vi "test Acyclic Loopback Selective Triggers.vi"(8 "error in":errorcluster, 11 "TestCase in":refnum<class "Single Board Loopback.lvclass">) -> (0 "error out":errorcluster, 3 "TestCase out":refnum<class "Single Board Loopback.lvclass">)   [LabVIEW 2020, in "Single Board Loopback.lvclass"]
uses:
  Single Board Loopback.lvclass
  <vilib>/addons/_JKI Toolkits/VI Tester/TestCase.llb/TestCase.lvclass
  <vilib>/NI VeriStand/Execution/Workspace/NI_VS Workspace ExecutionAPI.lvlib
  <vilib>/NI/VeriStand Custom Device Testing Tools/VeriStandTestUtilities/VeriStandTestUtilities.lvlib
  <vilib>/NI VeriStand/Execution/Workspace/NI VeriStand - Set Multiple Channel Values.vi
  <vilib>/numeric/Random Number (Range) U64.vi
  C:/Users/nitest/Desktop/Git 2020/niveristand-custom-device-testing-tools/VeriStandTestCase/VeriStandTestCase.lvclass
  C:/Program Files (x86)/National Instruments/LabVIEW 2020/vi.lib/addons/_JKI Toolkits/VI Tester/TestCase.llb/TestCase.lvclass
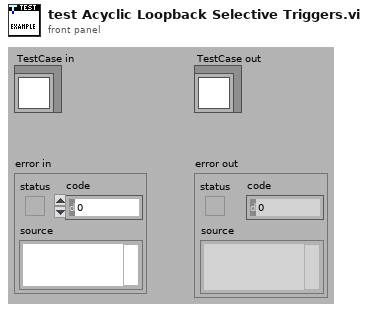
[diagram p1: front panel]
types:
  T1 = typedef "NI_VS Workspace ExecutionAPI.lvlib/WorkspaceAPI.ctl" = refnum<k24>
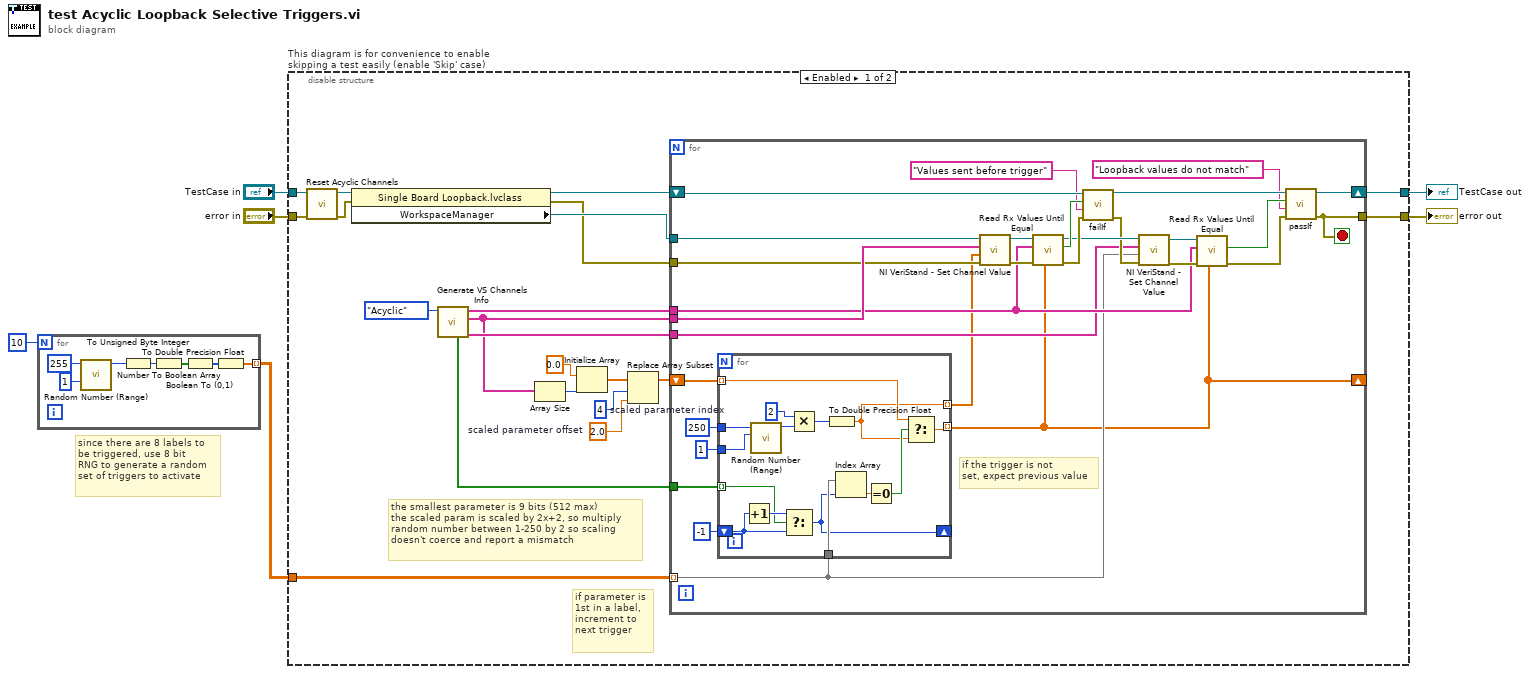
[diagram p0: block diagram]
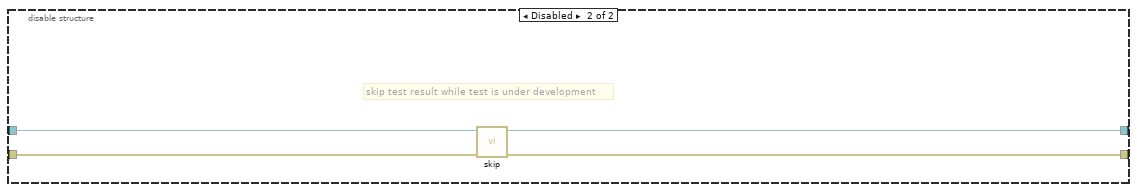
[diagram p2: hidden frame]
diagram:
  # "since there are 8 labels to\nbe triggered, use 8 bit \nRNG to generate a random\nset of triggers to activate"
  n1 = for {
    N: 10 -> [_]
    tunnel: [w7] -> w2 mode=indexing
    n2 = call-poly <vilib>:"Random Number (Range).vi"("lower bound (0)"=u64 1, "upper bound (100)"=u64 255) -> ("number"=w10:u64)  [unwired: 9 in]
    n3 = To Unsigned Byte Integer(number=w10) -> (unsigned 8bit integer=w9:u8)
    n4 = Number To Boolean Array(number=w9) -> (Boolean array=w13:bool[])
    n5 = Boolean To (0,1)(Boolean=w13) -> (0, 1=w8:i16[])
    n6 = To Double Precision Float(number=w8) -> (double precision float=w7:dbl[])
  }
  n7 = disable-structure "This diagram is for convenience to enable skipping a test easily (enable 'Skip' case)" shown="Enabled" {
    disable-tunnel: "TestCase in" -> [w14 w82]
    disable-tunnel: [w29 w80] -> w3
    disable-tunnel: [w28 w81] -> w5
    disable-tunnel: "error in" -> [w30 w79]
    disable-tunnel: w2 -> [w26 _]
    frame Enabled {
      w20 = 2.0  # scaled parameter offset
      w21 = 4  # scaled parameter index
      # "the smallest parameter is 9 bits (512 max)\nthe scaled param is scaled by 2x+2, so multiply \nrandom number between 1-250 by 2 so scaling\ndoesn't coerce and report a mismatch"
      # "if parameter is 1st in a label, increment to next trigger"
      n8 = call "Reset Acyclic Channels.vi"("error in (no error)"=w30, "reference in"=w14) -> ("error out"=w16:errorcluster, "reference out"=w15:refnum<class "Single Board Loopback.lvclass">)  [unwired: 8 in]
      n9 = property class="Single Board Loopback.lvclass"(reference=w15, error in=w16) -> (reference out=w31:refnum<class "Single Board Loopback.lvclass">, error out=w32:errorcluster, "WorkspaceManager"=w33:T1)
      n10 = call "Generate VS Channels Info.vi"("Transfer Type"=enum16{"Acyclic", "Scheduled"}."Acyclic") -> ("Tx Trigger Channels Array"=w27:string[], "Tx Channels Array"=w19:string[], "Rx Channels Array"=w34:string[], "Is First Parameter? Array"=w18:bool[])  [unwired: 6 in, 1 out]
      n11 = Array Size(array=w19) -> (size(s)=w24:i32)
      n12 = Initialize Array(0.0 ("element"), w24) -> (w25:dbl[])
      n13 = Replace Array Subset(array=w25, new element=w20, index=w21) -> (w22:dbl[])
      n14 = for {
        tunnel: w34 -> [w49]
        tunnel: w33 -> [w61]
        tunnel: w32 -> [w54]
        tunnel: w19 -> [w60]
        shift-right: [w45] -> w29
        shift-left: w31 -> [w56]
        tunnel: [w44] -> w28
        tunnel: w27 -> [w41]
        tunnel: w26 -> [w40] mode=indexing
        shift-right: [w37] -> _
        shift-left: w22 -> [w38]
        tunnel: w18 -> [w35]
        stop <- w44 stop-if-true
        # "if the trigger is not\nset, expect previous value"
        n15 = for {
          tunnel: [w68] -> w37 mode=indexing
          tunnel: u64 250 ("upper bound (100)") -> [w77]
          tunnel: u64 1 ("upper bound (100)") -> [w76]
          tunnel: w40 -> [w73]
          shift-right: [w72] -> _
          shift-left: -1 -> [w70]
          tunnel: w38 -> [w66] mode=indexing
          tunnel: [w65] -> w36 mode=indexing
          tunnel: w35 -> [w64] mode=indexing
          n16 = Increment(x=w70) -> (x+1=w71:i32)
          n17 = call-poly <vilib>:"Random Number (Range).vi"("lower bound (0)"=w76, "upper bound (100)"=w77) -> ("number"=w78:u64)  [unwired: 9 in]
          n18 = Select(t=w71, s=w64, f=w70) -> (s? t:f=w72:i32)
          n19 = Multiply(x=u64 2, y=w78) -> (x*y=w75:u64)
          n20 = To Double Precision Float(number=w75) -> (double precision float=w65:dbl)
          n21 = Index Array(array=w73, index=w72) -> (element=w69:dbl)
          n22 = Equal To 0?(x=w69) -> (x = 0?=w67:bool)
          n23 = Select(t=w66, s=w67, f=w65) -> (s? t:f=w68:dbl)
        }
        n24 = call-poly <vilib>:"NI VeriStand - Set Channel Value.vi"("error in (no error)"=w54, "Values"=w36, "Channels"=w60, "WorkspaceManager in"=w61) -> ("error out"=w57:errorcluster, "WorkspaceManager out"=w59:T1)  [unwired: 6 in]
        n25 = call <vilib>:"Read Rx Values Until Equal.vi"("expected values"=w37, "error in"=w57, "Rx aliases"=w49, "workspace manager in"=w59) -> ("error out"=w58:errorcluster, "values equal expected"=w55:bool, "workspace manager out"=w53:T1)  [unwired: 5 in]
        n26 = call-dynamic "failIf.vi"("error in (no error)"=w58, "message (\"\")"="Values sent before trigger" ("message (\"\")"), "fail"=w55, "TestCase in"=w56) -> ("error out"=w52:errorcluster, "TestCase out"=w46:refnum<class "Single Board Loopback.lvclass">)  [unwired: 6 in]
        n27 = call-poly <vilib>:"NI VeriStand - Set Channel Value.vi"("error in (no error)"=w52, "Values"=w40, "Channels"=w41, "WorkspaceManager in"=w53) -> ("error out"=w50:errorcluster, "WorkspaceManager out"=w51:T1)  [unwired: 6 in]
        n28 = call <vilib>:"Read Rx Values Until Equal.vi"("expected values"=w37, "error in"=w50, "Rx aliases"=w49, "workspace manager in"=w51) -> ("error out"=w47:errorcluster, "values equal expected"=w48:bool)  [unwired: 5 in, 1 out]
        n29 = call-dynamic "passIf.vi"("error in (no error)"=w47, "message (\"\")"="Loopback values do not match" ("message (\"\")"), "pass"=w48, "TestCase in"=w46) -> ("error out"=w44:errorcluster, "TestCase out"=w45:refnum<class "Single Board Loopback.lvclass">)  [unwired: 6 in]
      }
    }
    frame Disabled {
      # "skip test result while test is under development"
      n30 = call <vilib>:"skip.vi"("error in (no error)"=w79, "TestCase in"=w82) -> ("error out"=w81:errorcluster, "TestCase out"=w80:refnum<class "Single Board Loopback.lvclass">)  [unwired: 8 in]
    }
  }
  "error out" <- w5
  "TestCase out" <- w3
